vi "Throttle function FPGA.vi"(8 "RC input":i32, 11 "Channel 5 position":u8) -> (3 "Reference velocity":sgl)   [LabVIEW 2016]
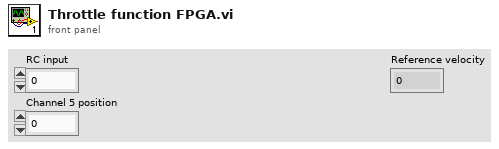
[diagram p1: front panel]
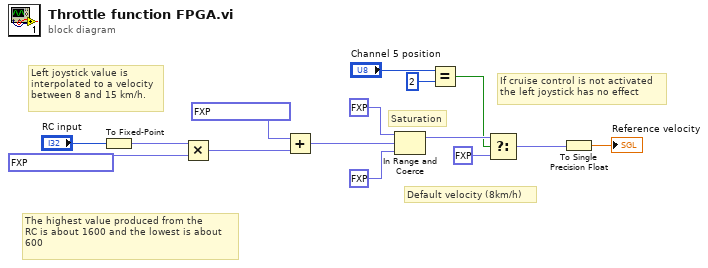
[diagram p0: block diagram]
diagram:
  # "The highest value produced from the\nRC is about 1600 and the lowest is about\n600"
  # "Default velocity (8km/h)"
  # "Saturation"
  # "If cruise control is not activated\nthe left joystick has no effect"
  # "Left joystick value is\ninterpolated to a velocity\nbetween 8 and 15 km/h."
  n1 = To Fixed-Point(number="RC input") -> (fixed-point=w14:fxp<+/-,32,32>)  [unwired: 1 in]
  n2 = Multiply(x=w14, y=fxp<+,16,1> 0.006988525390625 ("lower limit")) -> (x*y=w13:fxp<+/-,48,33>)
  n3 = Add(x=fxp<+/-,48,33> 3.79998779296875, y=w13) -> (x+y=w12:fxp<+/-,49,34>)
  n4 = In Range and Coerce(upper limit=fxp<+/-,33,33> 15.0, x=w12, lower limit=fxp<+/-,33,33> 8.0) -> (coerced(x)=w9:fxp<+/-,49,34>)  [unwired: 1 out]
  n5 = Equal?(x="Channel 5 position", y=u8 2) -> (x = y?=w8:bool)
  n6 = Select(t=w9, s=w8, f=fxp<+/-,49,34> 8.0) -> (s? t:f=w5:fxp<+/-,49,34>)
  n7 = To Single Precision Float(number=w5) -> (single precision float=→"Reference velocity":sgl)
